vi "Update HTML File.vi"(10 "Data In":T1, 11 "Path":path) -> (3 "URL out":string)   [LabVIEW 2016, in "Line Chart.xctl"]
uses:
  Line Chart.xctl
  Data Line Chart.ctl
panel:
  out "error out":errorcluster
  # "D:\\Ultratech\\Bitbucket\\Log Plotter\\xcontrol\\js"
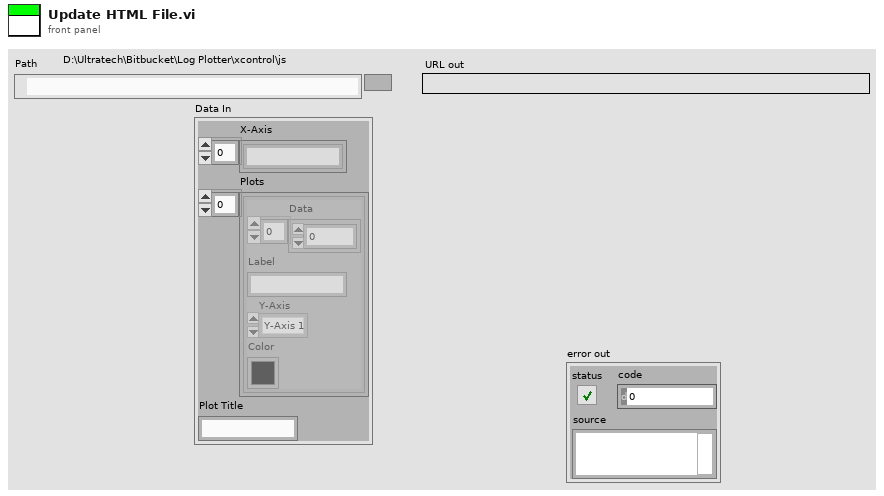
[diagram p1: front panel]
types:
  T1 = typedef "Line Chart.xctl/Data Line Chart.ctl" = cluster{"X-Axis":string[], "Plots":cluster{"Data":dbl[], "Label":string, "Y-Axis":enum16{"Y-Axis 1", "Y-Axis 2"}, "Color":u32}[], "Plot Title":string}
  T2 = enum16{"open", "replace", "create", "open or create", "replace or create", "replace or create with confirmation"}
  T3 = cluster{"Data":dbl[], "Label":string, "Y-Axis":enum16{"Y-Axis 1", "Y-Axis 2"}, "Color":u32}[]
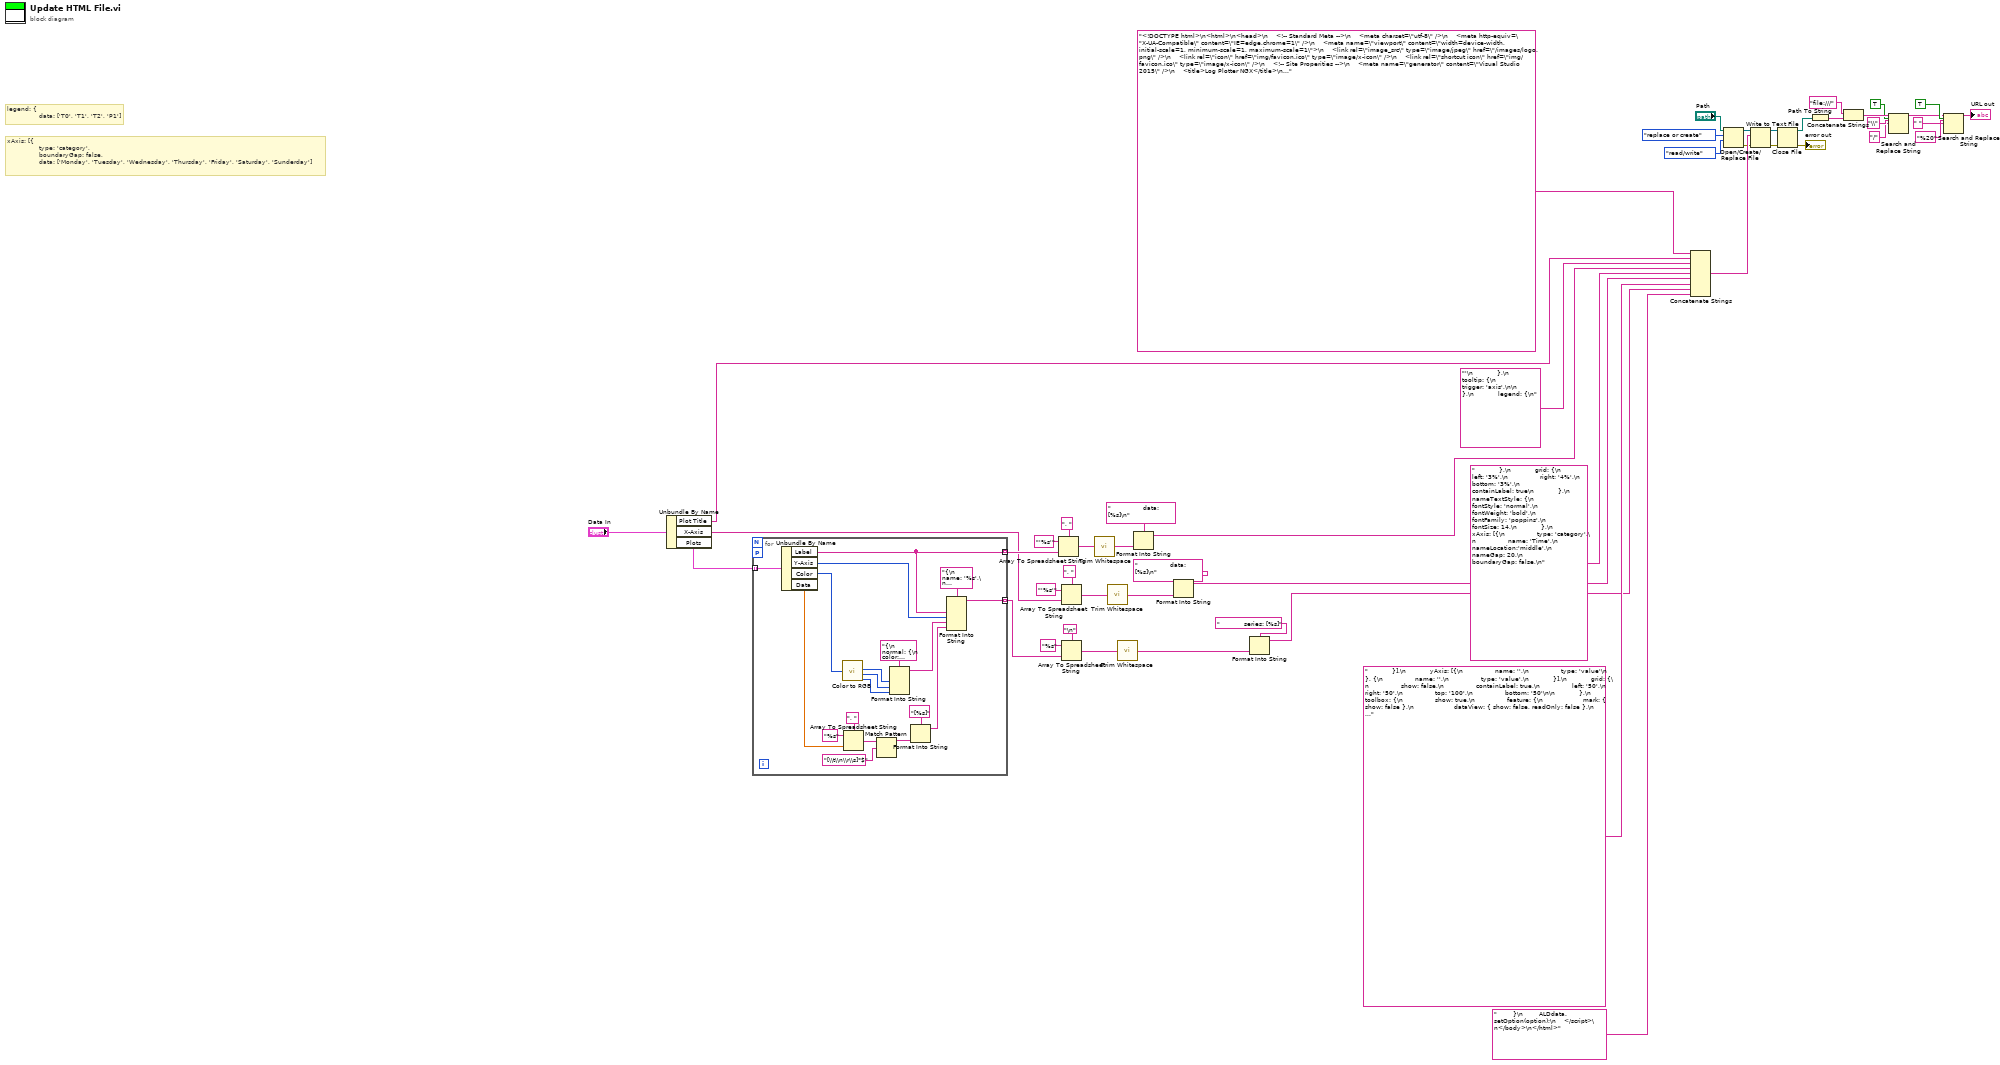
[diagram p0: block diagram]
diagram:
  # "xAxis: [{\n                type: 'category',\n                boundaryGap: false,\n                data: ['Monday', 'Tuesday', 'Wednesday', 'Thursday', 'Friday', 'Saturday', 'Sunderday']"
  # "legend: {\n                data: ['T0', 'T1', 'T2', 'P1']"
  n1 = Unbundle By Name("Data In") -> ("Plot Title"=w1:string, "X-Axis"=w44:string[], "Plots"=w50:T3)
  n2 = for {
    tunnel: w50 -> [w69] mode=indexing
    tunnel: [w59] -> w49 mode=indexing
    tunnel: [w56] -> w43 mode=indexing
    workers-P: _ -> [_]
    n3 = Unbundle By Name(w69) -> ("Label"=w59:string, "Y-Axis"=w58:enum16{"Y-Axis 1", "Y-Axis 2"}, "Color"=w65:u32, "Data"=w68:dbl[])
    n4 = call <vilib>:"Color to RGB.vi"("Color"=w65) -> ("R"=w63:u8, "G"=w62:u8, "B"=w61:u8)  [unwired: 1 out]
    n5 = Array To Spreadsheet String(delimiter (Tab)=", ", array=w68, 3:"%s" ("format string")) -> (spreadsheet string=w53:string)
    n6 = Match Pattern(string=w53, regular expression="[\\t\\n\\r\\s]*$") -> (before substring=w52:string)  [unwired: 1 in, 3 out]
    n7 = Format Into String(format string="{\n                    normal: {\n                        color: 'rgba(%d, %d,%d,10)',\n                            }\n                }", w63, w62, w61) -> (resulting string=w57:string)  [unwired: 2 in, 1 out]
    n8 = Format Into String(format string="[%s]", w52) -> (resulting string=w54:string)  [unwired: 2 in, 1 out]
    n9 = Format Into String(format string="{\n                name: '%s',\n                type: 'line',\n                yAxisIndex: %d,\n                smooth: true,\n                itemStyle:%s,\n                data:%s\n            },", w59, w58, w57, w54) -> (resulting string=w56:string)  [unwired: 2 in, 1 out]
  }
  n10 = Array To Spreadsheet String(delimiter (Tab)=", ", array=w49, 3:"'%s'" ("format string")) -> (spreadsheet string=w36:string)
  n11 = Array To Spreadsheet String(delimiter (Tab)=", ", array=w44, 3:"'%s'" ("format string")) -> (spreadsheet string=w33:string)
  n12 = Array To Spreadsheet String(delimiter (Tab)="\n", array=w43, 3:"%s" ("format string")) -> (spreadsheet string=w30:string)
  n13 = call <vilib>:"Trim Whitespace.vi"("string"=w36) -> ("trimmed string"=w28:string)  [unwired: 1 in]
  n14 = call <vilib>:"Trim Whitespace.vi"("string"=w33) -> ("trimmed string"=w27:string)  [unwired: 1 in]
  n15 = call <vilib>:"Trim Whitespace.vi"("string"=w30) -> ("trimmed string"=w26:string)  [unwired: 1 in]
  n16 = Format Into String(format string="                data: [%s]\n", w28) -> (resulting string=w35:string)  [unwired: 2 in, 1 out]
  n17 = Format Into String(format string="                data: [%s]\n", w27) -> (resulting string=w32:string)  [unwired: 2 in, 1 out]
  n18 = Format Into String(format string="            series: [%s]", w26) -> (resulting string=w29:string)  [unwired: 2 in, 1 out]
  n19 = Concatenate Strings("<!DOCTYPE html>\n<html>\n<head>\n    <!-- Standard Meta -->\n    <meta charset=\"utf-8\" />\n    <meta http-equiv=\"X-UA-Compatible\" content=\"IE=edge,chrome=1\" />\n    <meta name=\"viewport\" content=\"width=device-width, initial-scale=1, minimum-scale=1, maximum-scale=1\">\n    <link rel=\"image_src\" type=\"image/jpeg\" href=\"/images/logo.png\" />\n    <link rel=\"icon\" href=\"img/favicon.ico\" type=\"image/x-icon\" />\n    <link rel=\"shortcut icon\" href=\"img/favicon.ico\" type=\"image/x-icon\" />\n    <!-- Site Properities -->\n    <meta name=\"generator\" content=\"Visual Studio 2015\" />\n    <title>Log Plotter NGX</title>\n    <meta name=\"description\" content=\"Chartli Interactive Chart\" />\n    <meta name=\"keywords\" content=\"html5,chart,ui, library, framework, javascript,jquery,graphic,interactive\" />\n    <link href=\"css/semantic.css\" rel=\"stylesheet\" />\n    <link href=\"css/demo.css\" rel=\"stylesheet\" />\n</head>\n<body>\n\n<div id=\"ALD Data\" style=\"width: 100%;height:100%;\"></div>\n\n    <script src=\"js/jquery-2.1.4.min.js\"></script>\n    <script src=\"js/chartli.js\"></script>\n    <script>\n\n        var ALDdata = echarts.init(document.getElementById('ALD Data'));\n        option = {\n            backgroundColor: '#fffff',\n            color: ['#B33F62', '#F9564F', '#0C0A3E'],\n\n            title: {\n                text: '", w1, "'\n            },\n            tooltip: {\n                trigger: 'axis',\n\n            },\n            legend: {\n", w35, "            },\n            grid: {\n                left: '3%',\n                right: '4%',\n                bottom: '3%',\n                containLabel: true\n            },\n            nameTextStyle: {\n                fontStyle: 'normal',\n                fontWeight: 'bold',\n                fontFamily: 'poppins',\n                fontSize: 14,\n            },\n            xAxis: [{\n                type: 'category',\n                name: 'Time',\n                nameLocation:'middle',\n                nameGap: 20,\n                boundaryGap: false,\n", w32, "            }],\n            yAxis: [{\n                name: '',\n                type: 'value'\n            }, {\n                name: '',\n                type: 'value',\n            }],\n            grid: {\n                show: false,\n                containLabel: true,\n                left: '50',\n                right: '50',\n                top: '100',\n                bottom: '50'\n\n            },\n            toolbox: {\n                show: true,\n                feature: {\n                    mark: { show: false },\n                    dataView: { show: false, readOnly: false },\n                    magicType: { show: true, type: ['line', 'bar', 'stack', 'tiled'] },\n                    restore: { show: false, title: 'Refresh' },\n                    saveAsImage: { show: true, title: 'Save As Image' }\n                }\n            },\n            color: [\"#345995\", \"#03CEA4\", \"#FB4D3D\"],\n            dataZoom: {\n                show: true,\n                realtime: true,\n                start: 0,\n                end: 100\n            },\n", w29, "        }\n        ALDdata.setOption(option);\n    </script>\n</body>\n</html>") -> (w22:string)
  n20 = Open/Create/Replace File(file path (use dialog)="Path", operation (0:open)=T2."replace or create", access (0:read/write)=enum16{"read/write", "read-only", "write-only"}."read/write") -> (refnum out=w23:refnum<file>, error out=w16:errorcluster)  [unwired: 3 in, 1 out]
  n21 = Write to Text File(file (use dialog)=w23, text=w22, error in=w16) -> (refnum out=w20:refnum<file>, error out=w15:errorcluster)  [unwired: 1 in, 1 out]
  n22 = Close File(refnum=w20, error in=w15) -> (path=w17:path, error out=→"error out":errorcluster)
  n23 = Path To String(path=w17) -> (string=w19:string)
  n24 = Concatenate Strings("file:///" ("string"), w19) -> (w13:string)
  n25 = Search and Replace String(replace all?=TRUE ("replace all? (F)"), input string=w13, search string="\\", replace string="/" ("replace string (\"\")")) -> (result string=w6:string)  [unwired: 4 in, 3 out]
  n26 = Search and Replace String(replace all?=TRUE ("replace all? (F)"), input string=w6, search string=" ", replace string="%20" ("replace string (\"\")")) -> (result string=→"URL out":string)  [unwired: 4 in, 3 out]
